vi "Database.GetPrevStatus.vi"(7 "Idx":i32, 8 "error in":errorcluster, 9 "Serial":string[](array[string]), 10 "Refs":string[](array[string]), 11 "Data in":T1) -> (0 "error out":errorcluster, 2 "Status":i8, 3 "Data out":T1)   [LabVIEW 2016]
uses:
  Database.Data.ctl
  Database.Data.Status.ctl
  Database.Data.Sets.ctl
  Tools/EventLog/EventLog.EventSource.ctl
  Tools/EventLog/EventLog.EventLevel.ctl
  Tools/Translator/Translator.Message.ctl
  Tools/EventLog/EventLog.New(array).vi
  Global/ApplicationGlobal.vi
  Tools/EventLog/EventLog.Buffer.vi
  Tools/EventLog/EventLog.File.ReadWrite.vi
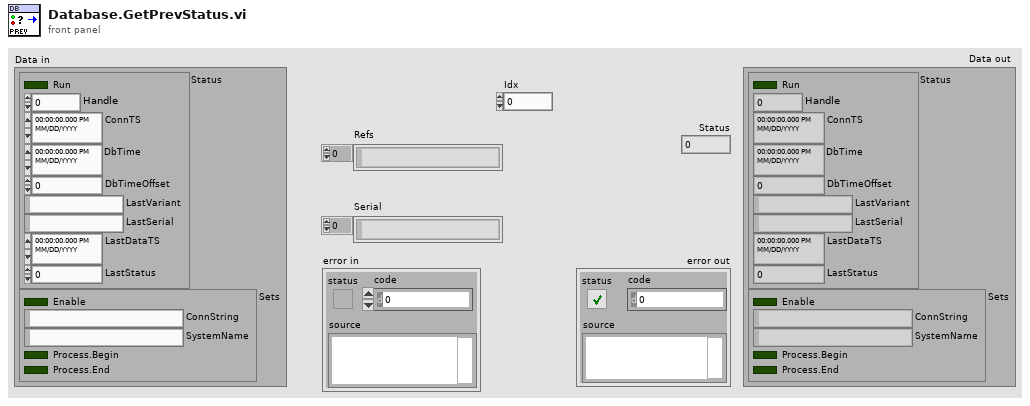
[diagram p1: front panel]
types:
  T1 = typedef "Database.Data.ctl" = cluster{"Status":T2, "Sets":T3}
  T2 = typedef "Database.Data.Status.ctl" = cluster{"Run":bool, "Handle":i32, "ConnTS":timestamp, "DbTime":timestamp, "DbTimeOffset":dbl, "LastVariant":string, "LastSerial":string, "LastDataTS":timestamp, "LastStatus":i32}
  T3 = typedef "Database.Data.Sets.ctl" = cluster{"Enable":bool, "ConnString":string, "SystemName":string, "Process.Begin":bool, "Process.End":bool}
  T4 = typedef "EventLog.EventSource.ctl" = enum16{"All", "Gui", "Cache", "PLC1", "PLC2", "PLC3", "DB", "DB01", "DB02", "DB03", "DB04", "DB05", "DB06", "DB07", "DB08", "DB09", "DB10", "DB11", "DB12", "DB13", "DB14", "DB15", "DB16"}
  T5 = typedef "Translator.Message.ctl" = enum16{"-", "Event confirmed", "Log out", "Log in", "Shutdown", "Cancel", "Start", "Continue", "Stop", "On", "Off", "OK", "NOK", "NOK %s", "This", "Prev", "Home", "Work", "In progress...", "Missing", "Empty", "Hardware failure", "Initial", "Error %d >> %s", "Error %d >> %s >> %s", "Starting %s", "Quitting %s", "Configured", "Initializing", "Quitting", "Loading", "Running %s", "Stopped", "Summary", "Do you want to continue?", "Do you want to exit?", "Log out?", "System", "All", "IDLE", "Translating...%s", "Not found", "Alarm %s", "Run", "Skip", "Abort", "Repeat", "Please wait...", "Database disconnected", "Login to database successful", "Login to database failed: %d; %s", "Get process step data for %s", "Changeover off", "Changeover into %s", "Product %s | %s found in cache with status %d at previous station", "Product %s | %s found in database with status %d at previous station", "Product %s | %s not found in cache at previous station", "Product %s | %s not found in database at previous station", "Product %s | %s found in cache with status %d at this station (%d repetion)", "Product %s | %s found in database with status %d at this station (%d repetition)", "Product %s | %s not found in cache at this station", "Product %s | %s not found in database at this station", "Product %s | %s found in cache for component %s | %s", "Product %s | %s found in database for component %s | %s", "Product not found in cache for component %s | %s", "Product not found in database for component %s | %s", "Product %s | %s connected with component %s | %s (cache)", "Product %s | %s connected with component %s | %s (database)", "New data for %s | %s (cache)", "New data for %s | %s (database)", "File %s moved (cache)", "File %s deleted (cache)", "Msg %d >> %s", "PLC LifeBit Failure", "Reconnecting DB", "Reconnecting PLC", "Free disk space is below 1GB - contact technician"}
  T6 = typedef "EventLog.EventLevel.ctl" = enum8{"Debug", "Info", "Warning", "Error"}
  T7 = typedef "Database.Data.Variant.Sets.ctl" = cluster{"PrevStations":string[], "ThisStations":string[]}
  T8 = typedef "ProdaNG.Identification.ctl" = cluster{"processId":i32, "systemId":i32, "processStepId":i32, "wabcoPartId":i32}
  T9 = typedef "ProdaNG.Product.ctl" = cluster{"c_id":string, "wabcoPartId":i32, "serialNumber":string, "comment":string, "individual":i32, "crProcessStepId":i32, "mdProcessStepId":i32, "crTime":string, "mdTime":string}
  T10 = typedef "ProdaNG.ProcessResult.ctl" = cluster{"c_id":string, "productId":string, "processId":i32, "statusId":i32, "startTime":string, "endTime":string}
  T11 = typedef "ProdaNG.ProcessStepResult.ctl" = cluster{"c_id":string, "processResultId":string, "processStepId":i32, "statusId":i32, "operatorId":i32, "startTime":string, "endTime":string}
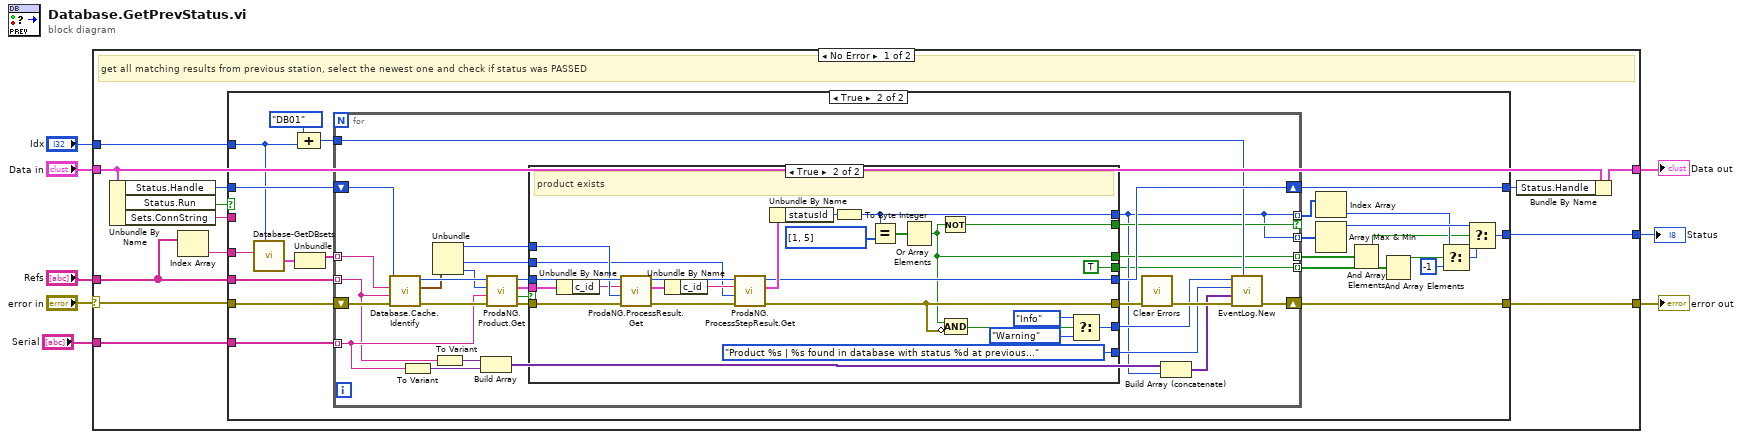
[diagram p0: block diagram]
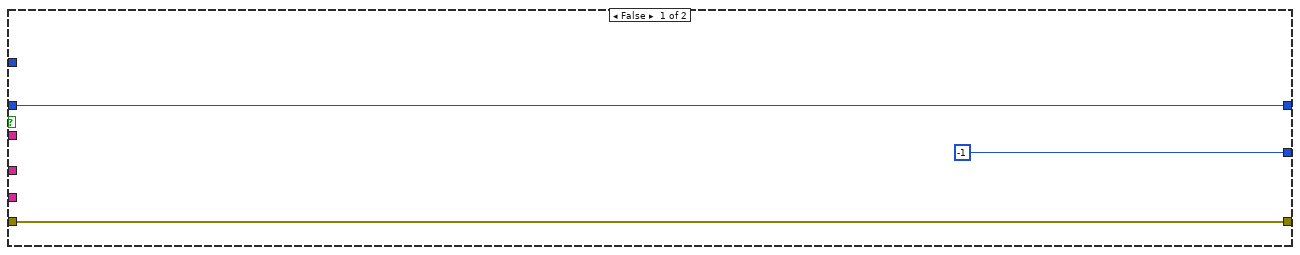
[diagram p2: hidden frame]
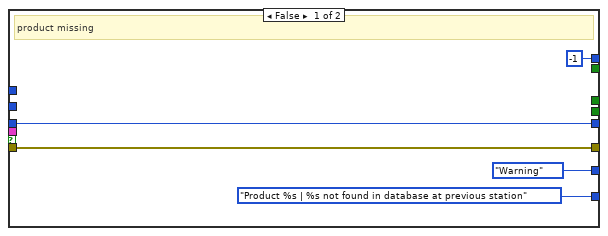
[diagram p3: hidden frame]
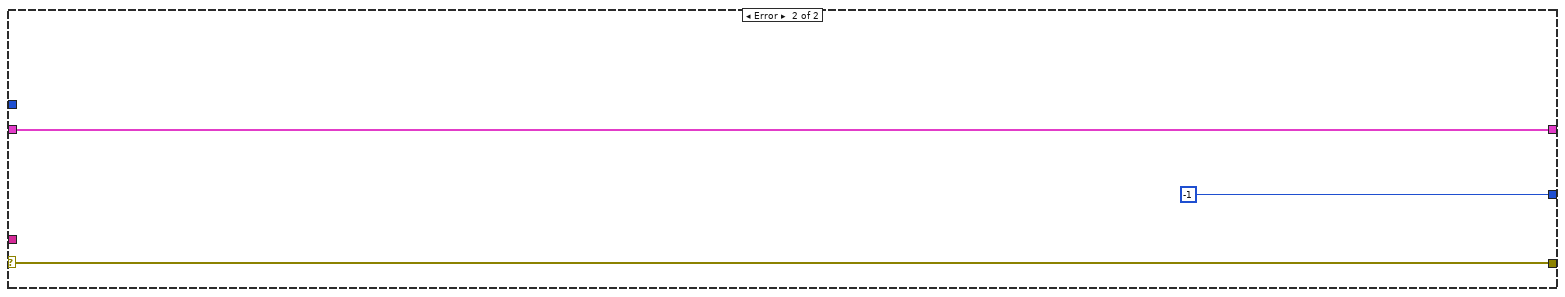
[diagram p4: hidden frame]
diagram:
  n1 = case shown="No Error" "error in" {
    selector: "error in" -> [w20 w110]
    tunnel: [w21 w110] -> w8
    tunnel: "Data in" -> [w18 w109]
    tunnel: [w17 w109] -> w5
    tunnel: "Idx" -> [w11 _]
    tunnel: "Serial" -> [w13 _]
    tunnel: "Refs" -> [w10 _]
    tunnel: [w12 i8 -1 ("f")] -> w3
    frame No Error {
      # "get all matching results from previous station, select the newest one and check if status was PASSED"
      n2 = Unbundle By Name(w18) -> ("Status.Handle"=w19:i32, "Status.Run"=w15:bool, "Sets.ConnString"=w14:string)
      n3 = Index Array(array=w10) -> (element=w9:string)  [unwired: 1 in]
      n4 = case shown="True" w15 {
        tunnel: w20 -> [w23 w45]
        tunnel: [w23 w26] -> w21
        tunnel: w19 -> [w24 w46]
        tunnel: [w24 w47] -> w16
        tunnel: w14 -> [_ _]
        tunnel: w13 -> [_ w42]
        tunnel: w10 -> [_ w43]
        tunnel: [i8 -1 ("f") w27] -> w12
        tunnel: w11 -> [_ w40]
        tunnel: w9 -> [_ w39]
        frame False {
        }
        frame True {
          n5 = call "Database-GetDBsets.vi"("Idx"=w40, "Variant"=w39) -> ("Variant Sets"=w41:T7)  [unwired: 5 in, 4 out]
          n6 = Unbundle(w41) -> ("PrevStations"=w25:string[])  [unwired: 1 out]
          n7 = Compound Arithmetic op=ADD(EventLog.EventSource."DB01" ("Source (All)"), w40) -> (w38:i32)
          n8 = for {
            tunnel: w42 -> [w53] mode=indexing
            shift-right: [w61] -> w26
            shift-left: w45 -> [w71]
            shift-right: [w63] -> w47
            shift-left: w46 -> [w69]
            tunnel: w43 -> [w52] mode=indexing
            tunnel: w25 -> [w64] mode=indexing
            tunnel: w38 -> [w60]
            tunnel: [w50] -> w31 mode=indexing if=w57
            tunnel: [w50] -> w32 mode=indexing
            tunnel: [w56] -> w30 mode=indexing
            tunnel: [w48] -> w29 mode=indexing
            n9 = call "Database.Cache.Identify.vi"("error in (no error)"=w71, "Variant"=w52, "SystemName"=w64, "DB Handle in"=w69) -> ("error out"=w72:errorcluster, "SytemID"=w68:T8, "DB Handle out"=w70:i32)  [unwired: 5 in]
            n10 = To Variant(anything=w53) -> (Variant=w55:variant)
            n11 = Unbundle(w68) -> ("processId"=w66:i32, "processStepId"=w65:i32, "wabcoPartId"=w67:i32)  [unwired: 1 out]
            n12 = To Variant(anything=w52) -> (Variant=w54:variant)
            n13 = Build Array(w54, w55) -> (w51:variant[])
            n14 = call "ProdaNG.Product.Get.vi"("error in (no error)"=w72, "serialNumber"=w53, "wabcoPartId"=w67, "dbHandle"=w70) -> ("error out"=w75:errorcluster, "found"=w73:bool, "Product"=w74:T9, "dbHandle out"=w76:i32)  [unwired: 4 in]
            n15 = case shown="True" w73 {
              tunnel: w75 -> [w82 w107]
              tunnel: [w82 w87] -> w77
              tunnel: w76 -> [w81 w105]
              tunnel: w74 -> [_ w106]
              tunnel: w66 -> [_ w104]
              tunnel: [w81 w97] -> w63
              tunnel: w65 -> [_ w96]
              tunnel: [Translator.Message."Product %s | %s not found in database at previous station" ("Message (-)") Translator.Message."Product %s | %s found in database with status %d at previous station" ("Message (-)")] -> w59
              tunnel: [EventLog.EventLevel."Warning" ("Level (Info)") w89] -> w58
              tunnel: [i8 -1 w86] -> w50
              tunnel: [_ w85] -> w57
              tunnel: [_ w84] -> w56
              tunnel: [_ TRUE] -> w48
              frame False {
                # "product missing"
              }
              frame True {
                # "product exists"
                n16 = Unbundle By Name(w106) -> ("c_id"=w98:string)
                n17 = call "ProdaNG.ProcessResult.Get.vi"("error in (no error)"=w107, "processId"=w104, "productId"=w98, "dbHandle"=w105) -> ("error out"=w101:errorcluster, "ProcessResult"=w103:T10, "dbHandle out"=w102:i32)  [unwired: 4 in, 1 out]
                n18 = Unbundle By Name(w103) -> ("c_id"=w99:string)
                n19 = call "ProdaNG.ProcessStepResult.Get.vi"("error in (no error)"=w101, "processStepId"=w96, "processResultId"=w99, "dbHandle"=w102) -> ("error out"=w87:errorcluster, "ProcessStepResult"=w100:T11, "dbHandle out"=w97:i32)  [unwired: 4 in, 1 out]
                n20 = Unbundle By Name(w100) -> ("statusId"=w93:i32)
                n21 = To Byte Integer(number=w93) -> (8bit integer=w86:i8)
                n22 = Equal?(x=w86, y=i8[] [1, 5]) -> (x = y?=w94:bool[])
                n23 = Or Array Elements(Boolean array=w94) -> (logical OR=w84:bool)
                n24 = Not(x=w84) -> (.not. x?=w85:bool)
                n25 = Compound Arithmetic op=AND(w84, invert w87) -> (w88:bool)
                n26 = Select(t=EventLog.EventLevel."Info" ("Level (Info)"), s=w88, f=EventLog.EventLevel."Warning" ("Level (Info)")) -> (s? t:f=w89:T6)
              }
            }
            n27 = call <vilib>:"Clear Errors.vi"("error in (no error)"=w77) -> ("error out"=w62:errorcluster)  [unwired: 5 in, 1 out]
            n28 = Build Array (concatenate)(w51, w50) -> (w49:variant[])
            n29 = call-poly "EventLog.New.vi"("Source (All)"=w60, "error in (no error)"=w62, "Arguments"=w49, "Message (-)"=w59, "Level (Info)"=w58) -> ("error out"=w61:errorcluster)  [unwired: 5 in, 1 out]
          }
          n30 = Index Array(array=w31) -> (element=w33:i8)  [unwired: 1 in]
          n31 = Array Max & Min(array=w32) -> (max value=w37:i8)  [unwired: 3 out]
          n32 = And Array Elements(Boolean array=w30) -> (logical AND=w28:bool)
          n33 = And Array Elements(Boolean array=w29) -> (logical AND=w36:bool)
          n34 = Select(t=w33, s=w36, f=i8 -1 ("max value")) -> (s? t:f=w34:i8)
          n35 = Select(t=w37, s=w28, f=w34) -> (s? t:f=w27:i8)
        }
      }
      n36 = Bundle By Name(cluster=w18, "Status.Handle"=w16) -> (w17:T1)
    }
    frame Error {
    }
  }
  "error out" <- w8
  "Data out" <- w5
  "Status" <- w3
